vi "Rio_X_Motor_PID_Speed_Control.vi"() -> ()   [LabVIEW 2017]
uses:
  <vilib>/myRIO/Common/Instrument Driver Framework/myRIO v1.0/Encoder/typedefs/Encoder Signal Mode.ctl
  <vilib>/myRIO/Instrument Drivers/Onboard IO/Encoder/typedefs/Encoder Reference.ctl
  <vilib>/myRIO/Common/Instrument Driver Framework/Utilities/typedefs/myRIO Generic Hardware Reference.ctl
  <vilib>/myRIO/Common/Instrument Driver Framework/Utilities/typedefs/Hardware Version Enum.ctl
  <vilib>/myRIO/Common/Instrument Driver Framework/Utilities/typedefs/myRIO v1.0 Reference.ctl
  <vilib>/myRIO/Common/Instrument Driver Framework/Utilities/typedefs/Generic FPGA Reference.ctl
  <vilib>/myRIO/Common/Instrument Driver Framework/myRIO v1.0/Encoder/typedefs/Encoder Channels Enum.ctl
  <vilib>/myRIO/Common/Instrument Driver Framework/myRIO v1.0/Encoder/typedefs/Encoder Configuration v1.0.ctl
  <vilib>/userdefined/High Color/nirio_resource_hc.ctl
  <vilib>/Analysis/1siggen.llb/Ramp Pattern by Samples.vi
  <vilib>/myRIO/Common/Instrument Driver Framework/Utilities/vis/Is FPGA Ref Available.vi
  <vilib>/myRIO/Common/Instrument Driver Framework/myRIO v1.0/Encoder/vis/myRIO v1.1 Open Encoder.vi
  <vilib>/myRIO/Instrument Drivers/Onboard IO/Encoder/vis/Read.vi
  <vilib>/myRIO/Common/Instrument Driver Framework/Utilities/vis/Validate Channels.vi
  <vilib>/myRIO/Common/Instrument Driver Framework/myRIO v1.0/Encoder/vis/myRIO v1.0 Reserve Encoder.vi
  <vilib>/myRIO/Common/Instrument Driver Framework/myRIO v1.0/Encoder/vis/myRIO v1.0 Build MUX Configuration Encoder.vi
  <vilib>/myRIO/Common/Instrument Driver Framework/myRIO v1.0/Resource Manager/vis/myRIO v1.0 Reserve Channel List.vi
  <vilib>/myRIO/Common/Instrument Driver Framework/myRIO v1.0/Resource Manager/vis/myRIO v1.0 Create Configuration List.vi
  <vilib>/myRIO/Common/Instrument Driver Framework/myRIO v1.0/Resource Manager/vis/myRIO v1.0 Reserve Channel.vi
  <vilib>/myRIO/Common/Instrument Driver Framework/myRIO v1.0/Resource Manager/vis/myRIO v1.0 Unreserve Channel.vi
  <vilib>/myRIO/Common/Instrument Driver Framework/myRIO v1.0/Resource Manager/vis/myRIO v1.0 Build Mutex Name.vi
  <vilib>/Utility/VariantDataType/GetNumericInfo.vi
  <vilib>/Utility/error.llb/Error Cluster From Error Code.vi
  <vilib>/myRIO/Common/Instrument Driver Framework/myRIO v1.0/myRIO v1.1 Open.vi
  <vilib>/myRIO/Common/Instrument Driver Framework/Utilities/vis/IO Manager.vi
  <vilib>/myRIO/Common/Instrument Driver Framework/Utilities/vis/Configuration Manager.vi
  <vilib>/myRIO/Common/Instrument Driver Framework/myRIO v1.0/Resource Manager/vis/myRIO v1.0 Configure IO.vi
  <vilib>/myRIO/Common/Instrument Driver Framework/myRIO v1.0/myRIO v1.0 Close.vi
  <vilib>/myRIO/Common/Instrument Driver Framework/myRIO v1.0/Encoder/vis/myRIO v1.0 Configure Encoder.vi
  <vilib>/myRIO/Common/Instrument Driver Framework/myRIO v1.0/Encoder/vis/myRIO v1.0 Read Encoder.vi
  <vilib>/addons/control/pid/pid.llb/PID (DBL).vi
  <vilib>/myRIO/Express VI/Onboard IO/Encoder/Encoder Express VI.xnode
  <vilib>/myRIO/Instrument Drivers/Onboard IO/Encoder/vis/myRIO Encoder Open.xnode
  <vilib>/myRIO/Common/Instrument Driver Framework/myRIO v1.0/Encoder/typedefs/Encoder Count Direction Enum.ctl
  <vilib>/myRIO/Instrument Drivers/Onboard IO/Encoder/Encoder.lvlib
  <vilib>/addons/control/pid/NI_PID_pid.lvlib
  <vilib>/Analysis/NI_AALBase.lvlib
panel:
  in  "s":bool
  out "Counter Value":i32
  out "element":dbl
  in  "Constant":dbl=500.0
  out "Waveform Graph":dbl[](graph)
  in  "Max V":dbl=100.0
  in  "End":dbl=200000.0
  in  "Start":dbl
  out "Error Out":errorcluster
  in  "Error In":errorcluster
  in  "Reset Counter":bool
  out "RPM Chart 2":cluster{"setpoint":dbl, dbl, "output":dbl}(graph)
  in  "PID gains":T1={"proportional gain (Kc)"=1.0, "integral time (Ti, min)"=0.01, "derivative time (Td, min)"=0.0} {"derivative time (Td, min)" format="%.3f"; "integral time (Ti, min)" format="%.3f"; "proportional gain (Kc)" format="%.3f"}
  in  "setpoint":dbl(slide) scale=-200.0..200.0
  out "RPM Chart":dbl(graph)
  in  "stop":bool
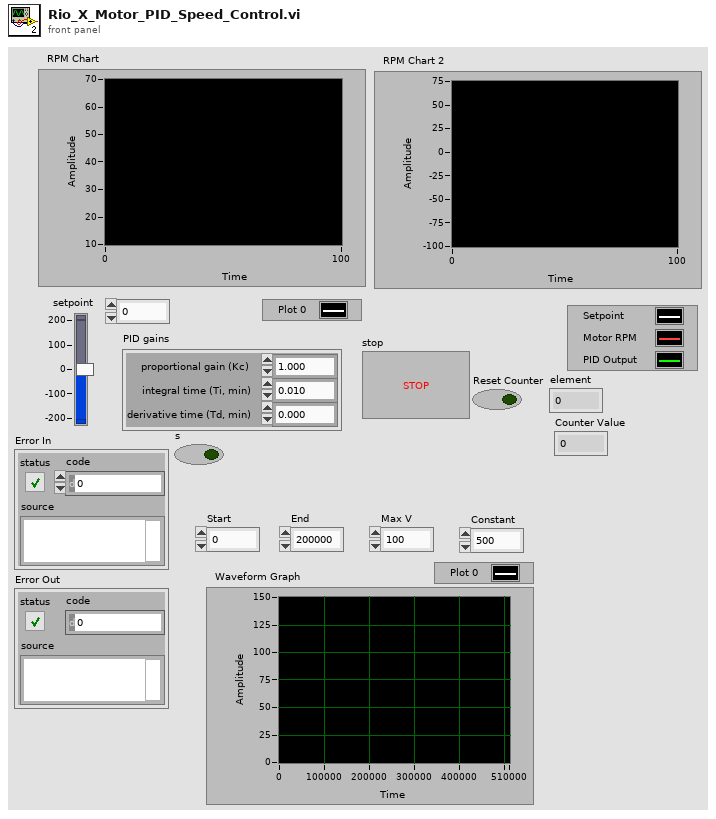
[diagram p1: front panel]
types:
  T1 = cluster{"proportional gain (Kc)":dbl, "integral time (Ti, min)":dbl, "derivative time (Td, min)":dbl}
  T2 = cluster{"X(t)/Y(f) Selection ":bool, "Duty Cycle (0-1) (X Control)":dbl, "Frequency [Hz] (Y Control)":dbl, "Direction (t:+, f:-)":bool}
  T3 = typedef "Encoder.lvlib/Encoder Reference.ctl" = cluster{"myRIO Reference":T4, "Encoder Channels Enum":T8}
  T4 = typedef "myRIO Generic Hardware Reference.ctl" = cluster{"myRIO Model":T5, "myRIO Hardware Reference":T6}
  T5 = typedef "Hardware Version Enum.ctl" = enum16{"Unknown", "myRIO-1900", "myRIO-1950", "roboRIO", "NI ELVIS RIO CM"}
  T6 = typedef "myRIO v1.0 Reference.ctl" = cluster{"Generic FPGA Reference":T7, "Allow multiple opens":bool}
  T7 = typedef "Generic FPGA Reference.ctl" = refnum<k20>
  T8 = typedef "Encoder Channels Enum.ctl" = enum16{"Not Connected", "C/ENC0", "C/ENC1", "A/ENC", "B/ENC", "DIO/ENC0", "DIO/ENC1", "DIO/ENC2", "DIO/ENC3", "DIO/ENC4"}
  T9 = typedef "Encoder Signal Mode.ctl" = enum16{"Quadrature phase signal", "Step and direction signal"}
  T10 = typedef "nirio_resource_hc.ctl" = tag
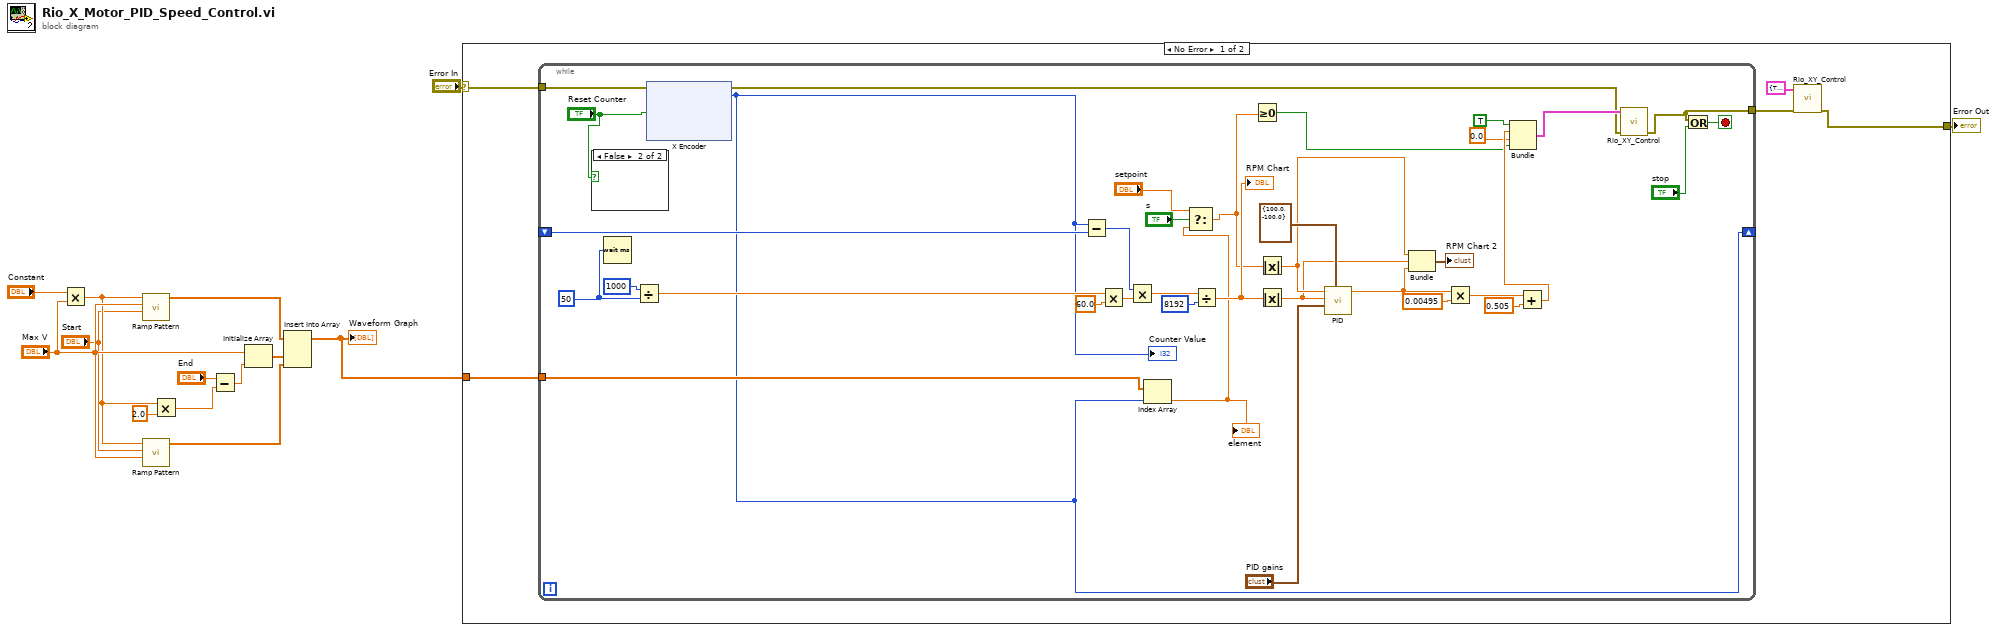
[diagram p0: block diagram]
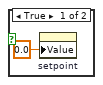
[diagram p2: hidden frame]
diagram:
  n1 = Multiply(x="Constant", y="Max V") -> (x*y=w10:dbl)
  n2 = call-poly <vilib>:"Ramp Pattern.vi"("start"="Start", "end"="Max V", "samples"=w10) -> ("Ramp Pattern"=w4:dbl[])  [unwired: 7 in, 1 out]
  n3 = call-poly <vilib>:"Ramp Pattern.vi"("start"="Max V", "end"="Start", "samples"=w10) -> ("Ramp Pattern"=w6:dbl[])  [unwired: 7 in, 1 out]
  n4 = Multiply(x=w10, y=2.0) -> (x*y=w9:dbl)
  n5 = Subtract(x="End", y=w9) -> (x-y=w8:dbl)
  n6 = Initialize Array("Max V", w8) -> (w5:dbl[])
  n7 = Insert Into Array(array=w4, new element #1=w5, new element #2=w6) -> (w1:dbl[])  [unwired: 1 in]
  "Waveform Graph" <- w1
  n8 = case shown="No Error" "Error In" {
    selector: "Error In" -> [w19 w103]
    tunnel: [w16 w103] -> w14
    tunnel: w1 -> [w15 _]
    frame No Error {
      n9 = while {
        shift-right: [w21] -> _
        shift-left: _ -> [w55]
        tunnel: [w29] -> w17
        tunnel: w19 -> [w36]
        tunnel: w15 -> [w22]
        stop <- w37 stop-if-true
        w28 = u32 50 ("milliseconds to wait")
        n10 = case shown="False" "Reset Counter" {
          frame True {
            n11 = property on="setpoint" class="Slide (strict)"("Value"=0.0 ("setpoint")) -> ()  [unwired: 2 in, 2 out]
          }
          frame False {
          }
        }
        n12 = Wait (ms)(milliseconds to wait=w28) -> ()  [unwired: 1 out]
        n13 = Divide(x=u32 1000, y=w28) -> (x/y=w40:dbl)
        n14 = xnode "X Encoder"("error in (no error)"=w36, "Reset Counter"="Reset Counter") -> ("error out"=w30:errorcluster, "Counter Value"=w21:i32)  [unwired: 2 out]
        "Counter Value" <- w21
        n15 = Subtract(x=w21, y=w55) -> (x-y=w53:i32)
        n16 = Multiply(x=w40, y=60.0) -> (x*y=w38:dbl)
        n17 = Multiply(x=w53, y=w38) -> (x*y=w52:dbl)
        n18 = Index Array(array=w22, index=w21) -> (element=w25:dbl)
        "element" <- w25
        n19 = Select(t="setpoint", s="s", f=w25) -> (s? t:f=w24:dbl)
        n20 = Divide(x=w52, y=8192) -> (x/y=w43:dbl)
        "RPM Chart" <- w43
        n21 = Greater Or Equal To 0?(x=w24) -> (x >= 0?=w32:bool)
        n22 = Absolute Value(x=w24) -> (abs(x)=w42:dbl)
        n23 = Absolute Value(x=w43) -> (abs(x)=w20:dbl)
        n24 = call-poly <vilib>:"PID.vi"("output range"=cluster{"output high":dbl, "output low":dbl} {"output high"=100.0, "output low"=-100.0}, "PID gains"="PID gains", "process variable"=w20, "setpoint"=w42) -> ("output"=w44:dbl)  [unwired: 6 in, 1 out]
        n25 = Bundle(w42, w20, "output"=w44) -> (→"RPM Chart 2":cluster{dbl, dbl, "output":dbl})  [unwired: 1 in]
        n26 = Multiply(x=w44, y=0.00495) -> (x*y=w47:dbl)
        n27 = Add(x=w47, y=0.505) -> (x+y=w34:dbl)
        n28 = Bundle(TRUE, w34, 0.0, w32) -> (w31:cluster{bool, dbl, dbl, bool})  [unwired: 1 in]
        n29 = call "Rio_XY_Control.vi"("Error In"=w30, "Input Cluster"=w31) -> ("Error Out"=w29:errorcluster)  [unwired: 9 in]
        n30 = Or(x=w29, y="stop") -> (x .or. y?=w37:bool)
      }
      n31 = call "Rio_XY_Control.vi"("Error In"=w17, "Input Cluster"=T2 {"X(t)/Y(f) Selection "=TRUE, "Duty Cycle (0-1) (X Control)"=0.0, "Frequency [Hz] (Y Control)"=0.0, "Direction (t:+, f:-)"=TRUE}) -> ("Error Out"=w16:errorcluster)  [unwired: 9 in]
    }
    frame Error {
    }
  }
  "Error Out" <- w14
